vi "运维调试_总磷氨氮.vi"() -> ()   [LabVIEW 2016, in "斯坦道仪器.lvlib"]
uses:
  <vilib>/Platform/TimedLoop/XDataNode/timing_clust.ctl
  <vilib>/Platform/TimedLoop/XDataNode/nitl_modes.ctl
  <vilib>/Platform/TimedLoop/XDataNode/wakeup.ctl
  <vilib>/Utility/miscctls.llb/LVPointTypeDef.ctl
  <vilib>/Platform/TimedLoop/XDataNode/XDataNode.xnode
  <vilib>/Platform/TimedLoop/XDataNode/XDNodeRunTimeDep.lvlib
panel:
  out "固件版本号":string
  in  "参数":T1={"站号"=3, "量程切换"=enum."AUTO", "控制命令"=enum."启动测量", "模式设置"=enum."待机", "测量间隔"=0} {"站号" items=["氨氮"=3]}
  out "error out":errorcluster
  in  "同步时间":bool
  in  "数组":string[](array[string])
  in  "备用系数写入":bool
  in  "备用系数读取":bool
  in  "备用系数":T2
  in  "量程切换阈值写入":bool
  in  "量程切换阈值读取":bool
  in  "量程切换阈值":cluster{"阈值":dbl, "标液浓度":dbl}
  in  "参数下拉列表":enum16{"氨氮"}(ring)
  in  "量程下拉列表":enum16{"低量程", "高量程"}(ring)
  in  "测量模式下拉列表":enum16{"水样测量", "空白核查", "标样核查", "盲样测试", "加标回收"}(ring)
  in  "公式":cluster{"X^2":dbl, "X":dbl, "b":dbl}
  in  "写公式":bool
  in  "读公式":bool
  in  "精度":dbl=4.0
  in  "样品5 F0":dbl
  in  "样品5 F1":dbl
  in  "样品4 F1":dbl
  in  "样品4 F0":dbl
  in  "样品3 F0":dbl
  in  "样品3 F1":dbl
  in  "样品2 F0":dbl
  in  "样品2 F1":dbl
  in  "样品1 F1":dbl
  in  "样品1 F0":dbl
  in  "method":u16(ring) items=["最小二乘", "最小绝对残差", "Bisquare"]
  in  "模型":enum32{"线性", "多项式"}(ring)
  out "r^2":dbl format="%.7g"
  out "拟合公式":string
  in  "样品2启用":bool
  in  "样品5启用":bool
  in  "样品4启用":bool
  in  "样品3启用":bool
  in  "样品1启用":bool
  in  "标液浓度5":dbl
  out "测量吸光度5":dbl
  in  "标液浓度4":dbl
  out "测量吸光度4":dbl
  in  "标液浓度3":dbl
  out "测量吸光度3":dbl
  in  "标液浓度2":dbl
  out "测量吸光度2":dbl
  out "测量吸光度1":dbl
  in  "标液浓度1":dbl
  out "XY图":cluster{"X Values":dbl[], "Y Values":dbl[]}[](graph)
  in  "返回":bool
  in  "设置":bool
  out "序列号":string="序列号"
  out "氨氮测量数据":T3(xcontrol)
  out "总磷测量数据":T3(xcontrol)
  out "集成报警信息":string
  out "设置值":dbl
  out "定时启动":bool
  out "总磷总氮运行状态":T4(xcontrol)
  in  "停止":bool
  in  "手动启动":bool
  in  "单步测试":bool
  in  "总磷氨氮调试":u16[](xcontrol)
  out "F3":sgl format="%#.6f"
  out "F2":sgl format="%#.6f"
  out "F1":sgl format="%#.6f"
  out "F0":sgl format="%#.6f"
  out "多列列表框":i32(listbox)
  # "COM4"
  # "参数设置"
  # "标液浓度"
  # "F0"
  # "F1"
  # "吸光值显示"
  # "样品一"
  # "辅\n助\n计\n算\n区"
  # "样品二"
  # "样品三"
  # "样品四"
  # "样品五"
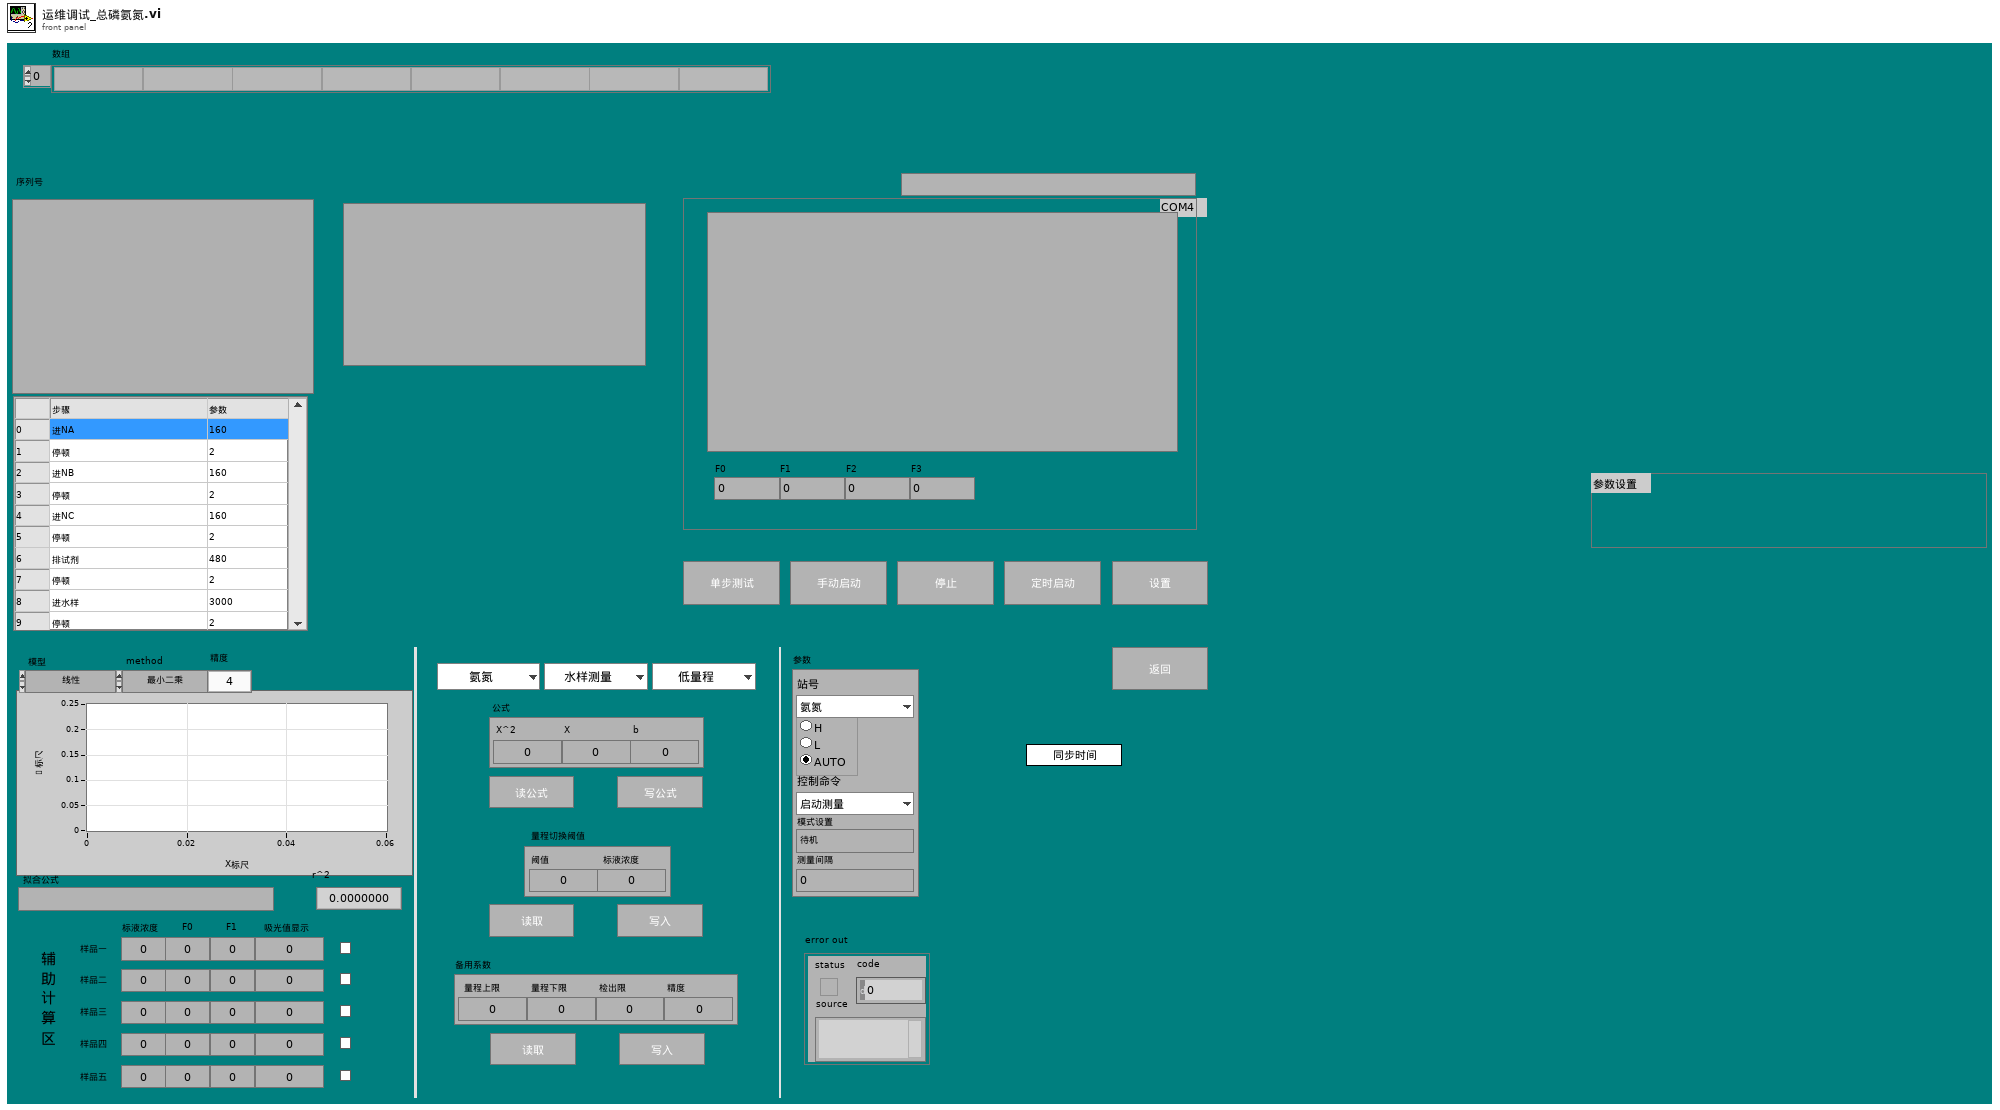
[diagram p1: front panel]
types:
  T1 = cluster{"站号":u16, "量程切换":enum32{"H", "L", "AUTO"}, "控制命令":enum16{"启动测量", "标样核查", "零点核查", "跨度核查", "空白测试", "平行样测试", "加标回收", "空白校准", "标样校准", "初始化（清洗）", "停止测试", "仪器重启", "校时", "模式设置", "测量间隔设置", ""}, "模式设置":enum16{"待机", "连续模式", "周期模式", "定点模式", "受控模式", "手动模式"}, "测量间隔":u16}
  T2 = cluster{"量程上限":dbl, "量程下限":dbl, "检出限":dbl, "精度":dbl}
  T3 = cluster{"flowid":u16, "测量精度":u16, "测量数据区":cluster{"因子编码":u32, "单位":u16, "标样参考值":sgl, "水样数据时间":timestamp, "水样实测值":sgl, "水样数据标识":string, "标样数据时间":timestamp, "标样实测值":sgl, "标样数据标识":string, "空白数据时间":timestamp, "空白实测值":sgl, "空白数据标识":string, "零点核查数据时间":timestamp, "零点核查实测值":sgl, "零点核查数据标识":string, "跨度核查数据时间":timestamp, "跨度核查实测值":sgl, "跨度核查数据标识":string, "加标回收数据时间":timestamp, "加标回收实测值":sgl, "加标回收数据标识":string, "平行样数据时间":timestamp, "平行样实测值":sgl, "平行样数据标识":string}}
  T4 = cluster{"系统时间":timestamp, "工作状态":enum16{"空闲", "水样测试", "标样核查", "零点核查", "跨度核查", "空白测试", "平行样测试", "加标回收", "空白校准", "标样校准", "初始化（清洗）"}, "测量模式":enum16{"待机", "连续模式", "周期模式", "定点模式", "受控模式", "手动模式"}, "告警代码":enum16{"无告警", "缺试剂告警", "缺水样告警", "缺蒸馏水告警", "缺标液告警", "仪表漏液告警", "标定异常告警", "超量程告警", "加热异常", "低试剂预警", "超上限告警", "超下限告警", "仪表内部其他异常", "滴定异常告警", "电极异常告警", "量程切换告警", "参数设置告警", "PH电极电位异常", "电导率电极异常", "浊度光度异常", "溶解氧电极异常", "溶解氧光强异常", "温度异常告警", "PH异常告警", "溶解氧异常告警", "电导率异常告警", "浊度异常告警", "叶绿素异常告警", "藻密度异常告警", "蓝绿藻异常告警", "ORP异常告警", "氨氮异常告警", "清洁刷异常告警", "SD卡异常告警", "蓝牙异常告警", "Wifi异常告警", "流程异常告警"}, "故障代码":enum16{"无故障", "电机故障", "温度故障", "通讯故障", "滴定故障"}, "日志代码":u16, "软件版本":u16, "F0":sgl, "F1":sgl, "F2":sgl, "F3":sgl, "T":sgl, "H":sgl, "id":u16, "flowid":u16, "量程":u16}
  T5 = enum16{"待机", "启动氨氮", "氨氮测量中", "启动总磷", "总磷测量中", "延时"}
  T6 = typedef "LVPointTypeDef.ctl" = cluster{"Horizontal":i16, "Vertical":i16}
  T7 = cluster{"因子编码":u32, "单位":u16, "标样参考值":sgl, "水样数据时间":timestamp, "水样实测值":sgl, "水样数据标识":string, "标样数据时间":timestamp, "标样实测值":sgl, "标样数据标识":string, "空白数据时间":timestamp, "空白实测值":sgl, "空白数据标识":string, "零点核查数据时间":timestamp, "零点核查实测值":sgl, "零点核查数据标识":string, "跨度核查数据时间":timestamp, "跨度核查实测值":sgl, "跨度核查数据标识":string, "加标回收数据时间":timestamp, "加标回收实测值":sgl, "加标回收数据标识":string, "平行样数据时间":timestamp, "平行样实测值":sgl, "平行样数据标识":string}
  T8 = enum16{"空闲", "水样测试", "标样核查", "零点核查", "跨度核查", "空白测试", "平行样测试", "加标回收", "空白校准", "标样校准", "初始化（清洗）"}
  T9 = cluster{"启动模式":enum16{"标液测量", "水样测量", "零液测量", "盲样测量", "加标回收"}, "启动参数":u16, "量程":enum16{"低量程", "高量程"}}
  T10 = cluster{"时间标识":timestamp, "设备":string, "日志信息":string, "流程参数":string}
  T11 = cluster{"时间标识":timestamp, "设备":string, "日志信息":string}
  T12 = enum16{"无告警", "缺试剂告警", "缺水样告警", "缺蒸馏水告警", "缺标液告警", "仪表漏液告警", "标定异常告警", "超量程告警", "加热异常", "低试剂预警", "超上限告警", "超下限告警", "仪表内部其他异常", "滴定异常告警", "电极异常告警", "量程切换告警", "参数设置告警", "PH电极电位异常", "电导率电极异常", "浊度光度异常", "溶解氧电极异常", "溶解氧光强异常", "温度异常告警", "PH异常告警", "溶解氧异常告警", "电导率异常告警", "浊度异常告警", "叶绿素异常告警", "藻密度异常告警", "蓝绿藻异常告警", "ORP异常告警", "氨氮异常告警", "清洁刷异常告警", "SD卡异常告警", "蓝牙异常告警", "Wifi异常告警", "流程异常告警"}
  T13 = typedef "LVRowAndColumnUnsignedTypeDef.ctl" = cluster{"Row":u32, "Column":u32}
  T14 = typedef "XDNodeRunTimeDep.lvlib/timing_clust.ctl" = cluster{"Expected End [f-1]":u64, "Actual End [f-1]":u64, "Finished Late? [f-1]":bool, "Expected End [i-1]":u64, "Actual End [i-1]":u64, "Finished Late? [i-1]":bool, "Expected Start [i]":u64, "Actual Start [i]":u64, "Expected Start [f]":u64, "Actual Start [f]":u64, "Source Name":string, "Structure Name":string, "Period":i64, "Deadline":i64, "Offset":i64, "Start":i64, "Priority":i32, "Timeout":i32, "Mode":T15, "Wakeup Reason":T16, "Error":errorcluster, "Source Type":string, "Secondary Source Type":string, "Global End Time":u64, "Global Start Time":u64, "Frame Duration":u64, "Iteration Duration":u64, "Assigned CPU":i32, "I/O Scan Engine Mode":u32}
  T15 = typedef "XDNodeRunTimeDep.lvlib/nitl_modes.ctl" = enum32{"No Change", "Process missed periods, maintain original phase", "Discard missed periods, maintain original phase", "Process missed periods, ignore original phase", "Discard missed periods, ignore original phase"}
  T16 = typedef "XDNodeRunTimeDep.lvlib/wakeup.ctl" = enum32{"Normal", "Aborted", "Asynchronous wakeup", "Timing source error", "Timed loop error", "Timeout"}
  T17 = cluster{"站号":u16, "量程切换":enum32{"H", "L", "AUTO"}, "控制命令":enum16{"启动测量", "标样核查", "零点核查", "跨度核查", "空白测试", "平行样测试", "加标回收", "空白校准", "标样校准", "初始化（清洗）", "停止测试", "仪器重启", "校时", "模式设置", "测量间隔设置", "盲样测试"}, "模式设置":enum16{"待机", "连续模式", "周期模式", "定点模式", "受控模式", "手动模式"}, "测量间隔":u16}
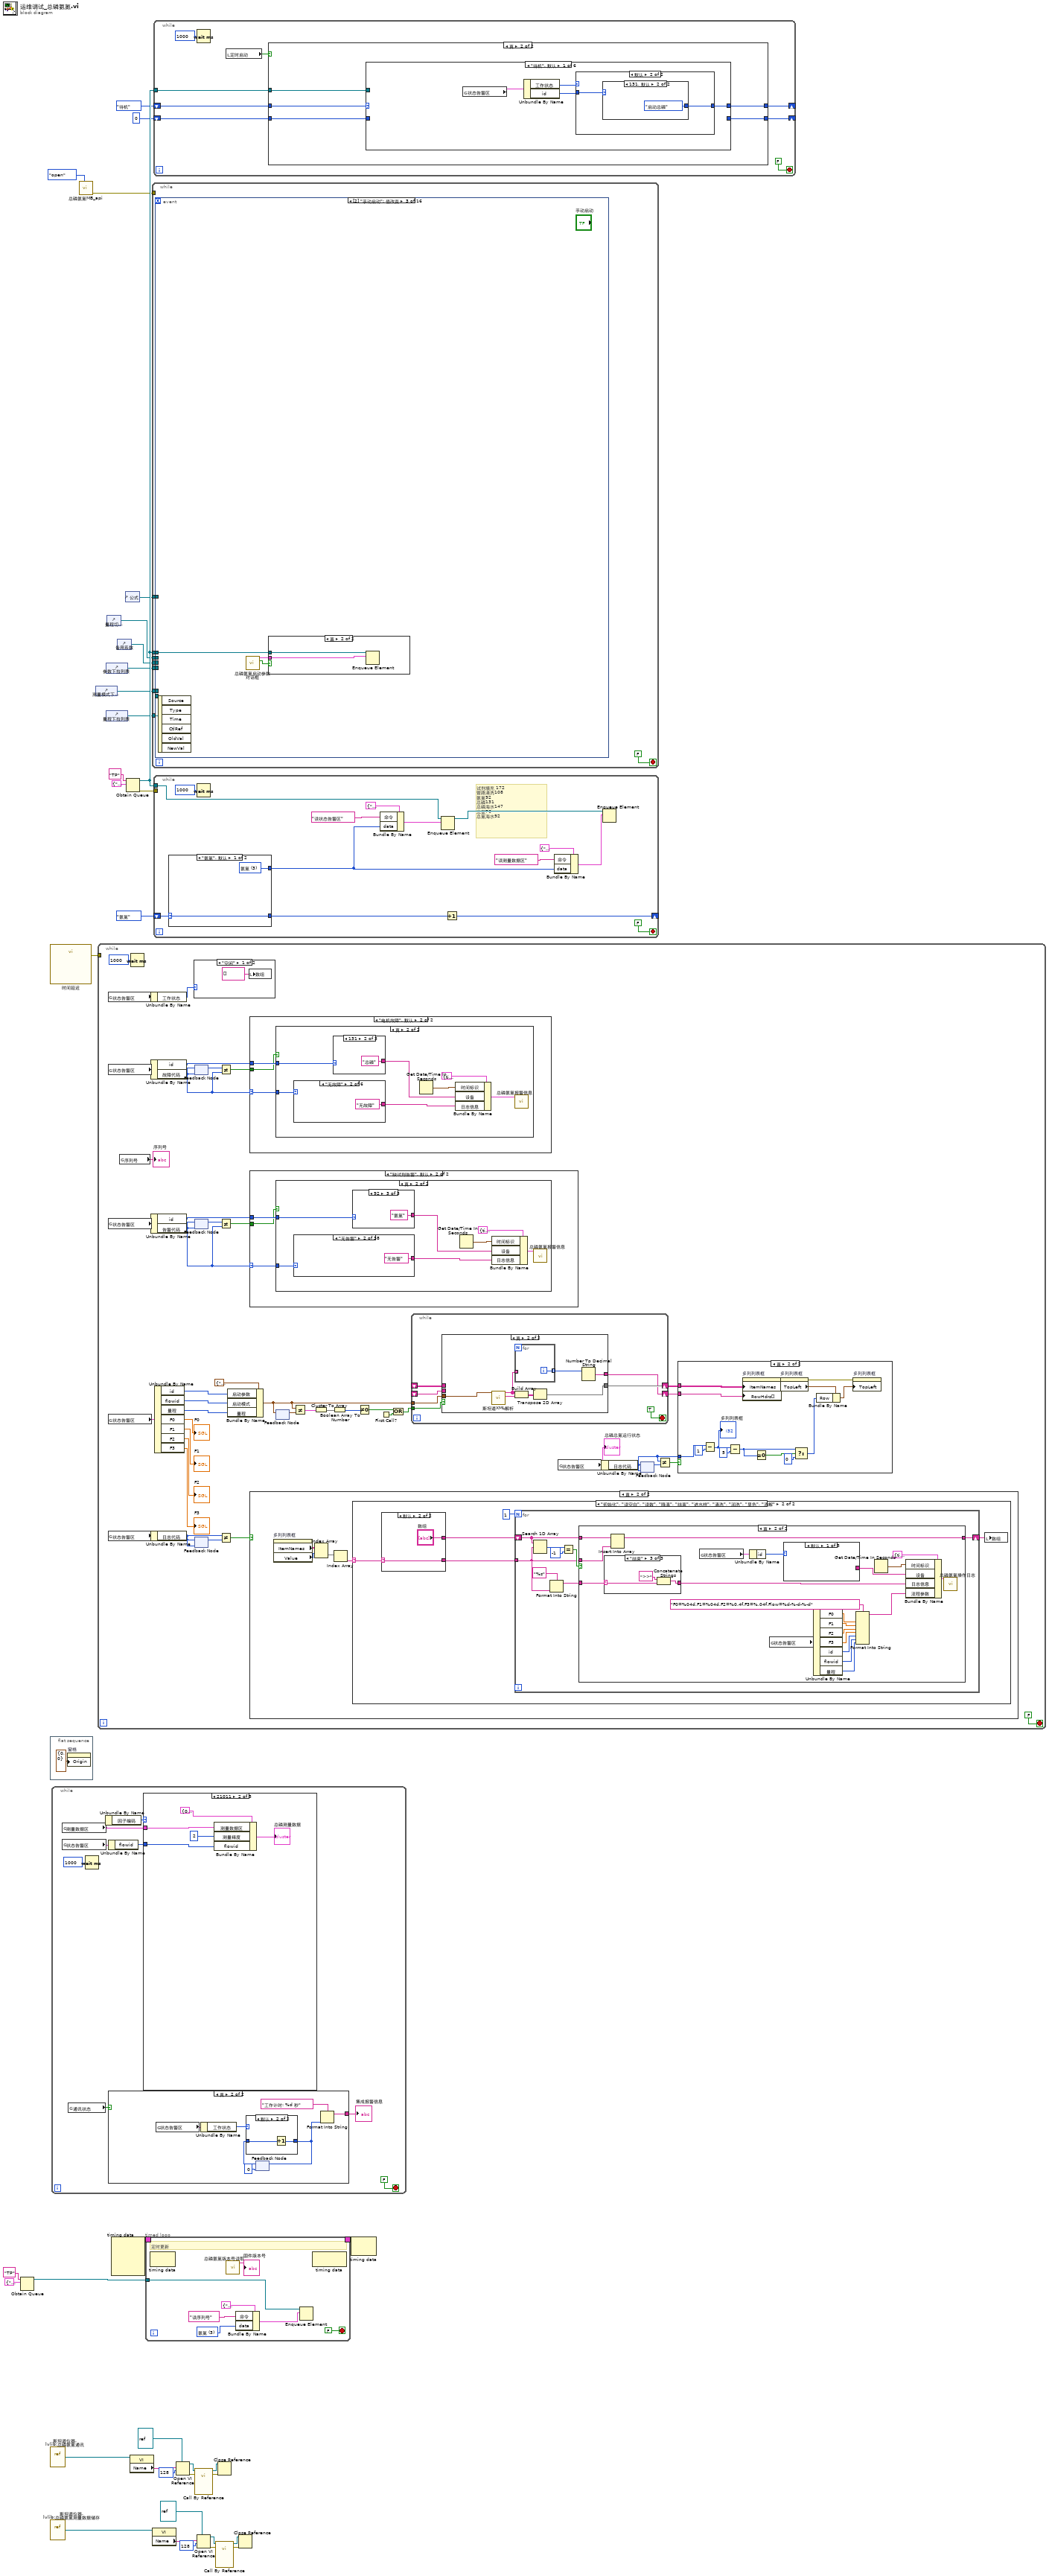
[diagram p0: block diagram]
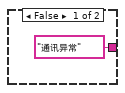
[diagram p2: hidden frame]
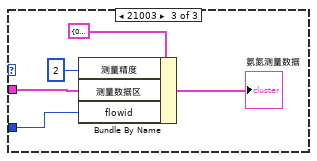
[diagram p5: hidden frame]
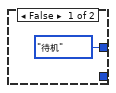
[diagram p6: hidden frame]
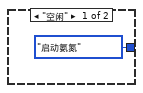
[diagram p7: hidden frame]
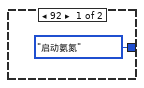
[diagram p8: hidden frame]
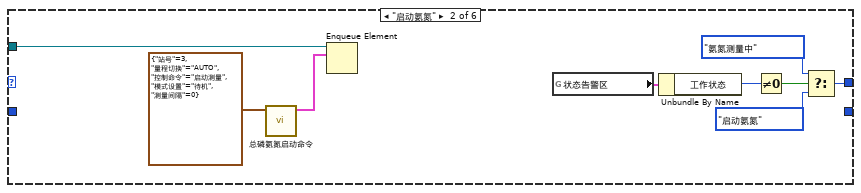
[diagram p9: hidden frame]
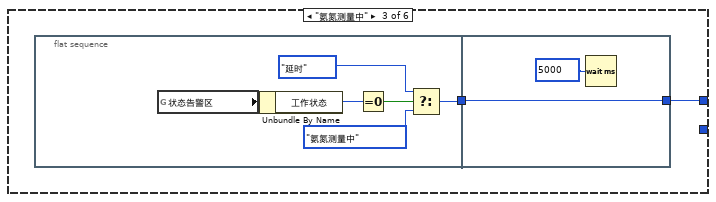
[diagram p10: hidden frame]
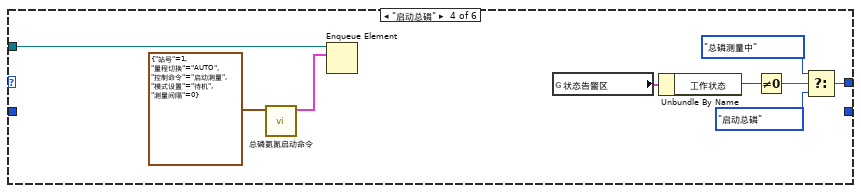
[diagram p11: hidden frame]
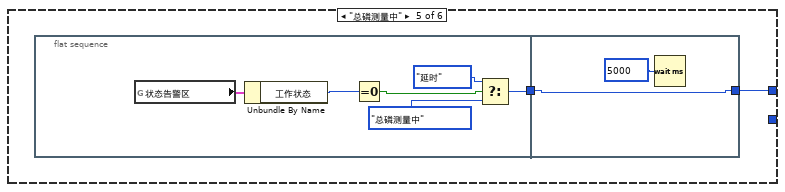
[diagram p12: hidden frame]
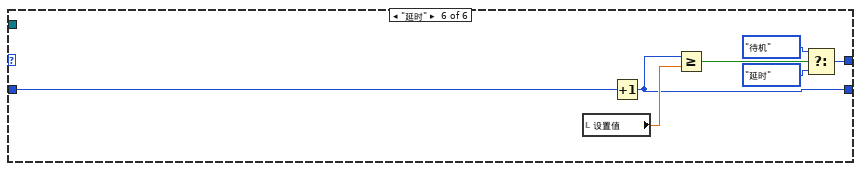
[diagram p13: hidden frame]
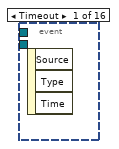
[diagram p14: hidden frame]
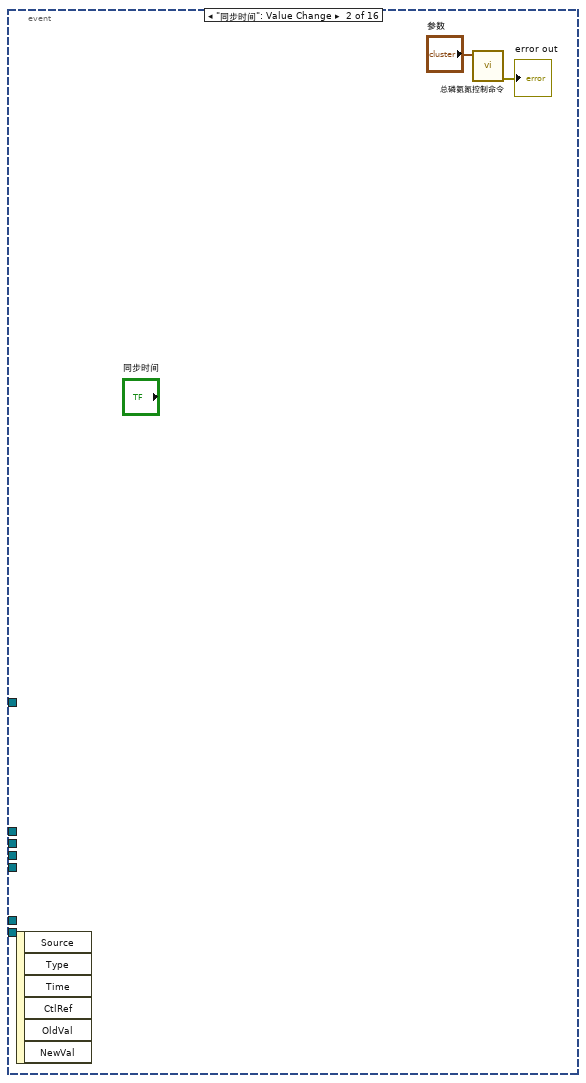
[diagram p15: hidden frame]
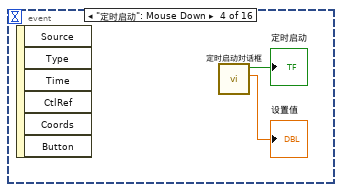
[diagram p17: hidden frame]
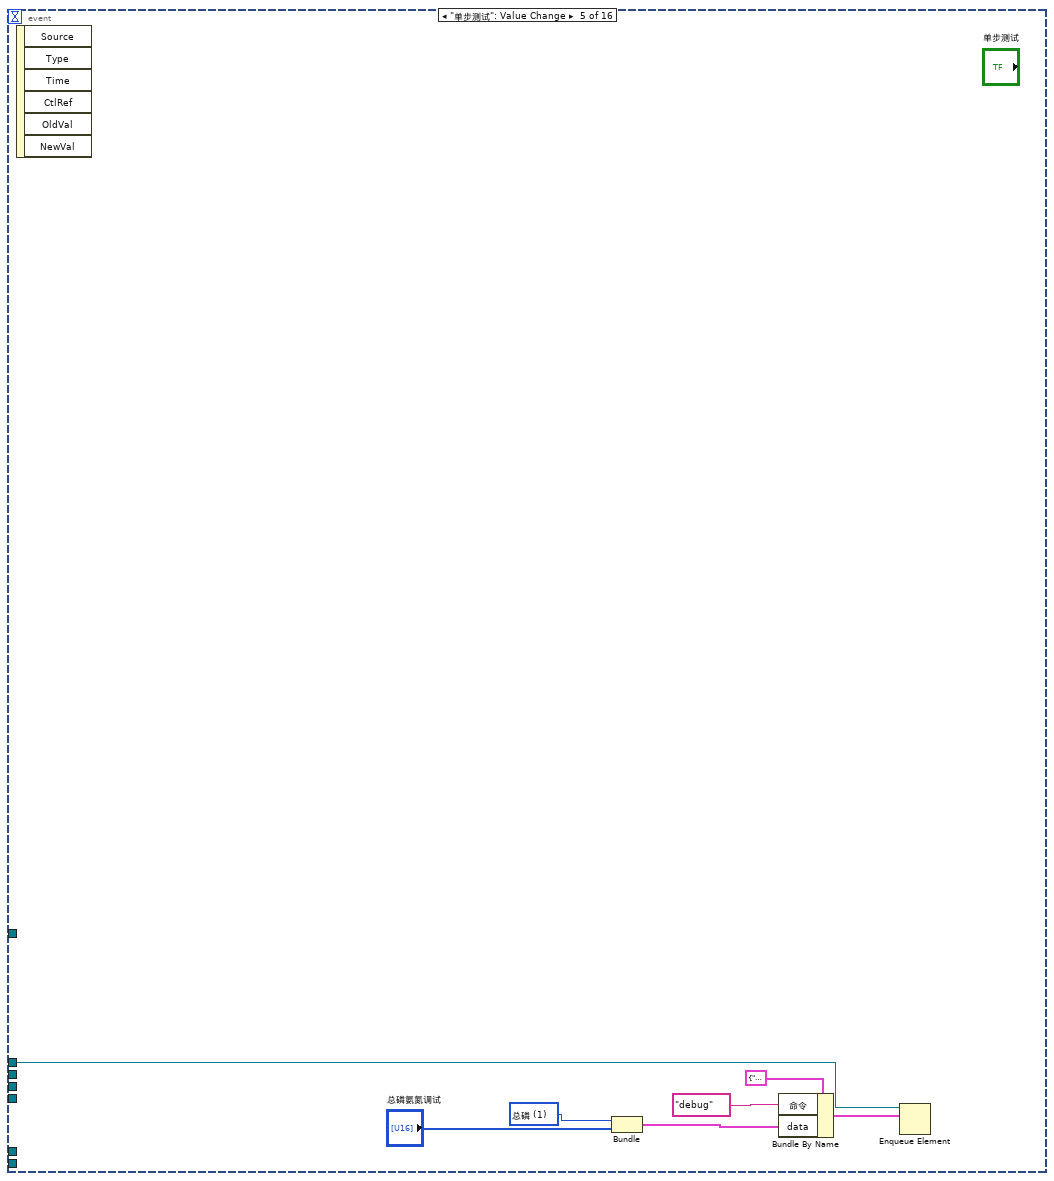
[diagram p18: hidden frame]
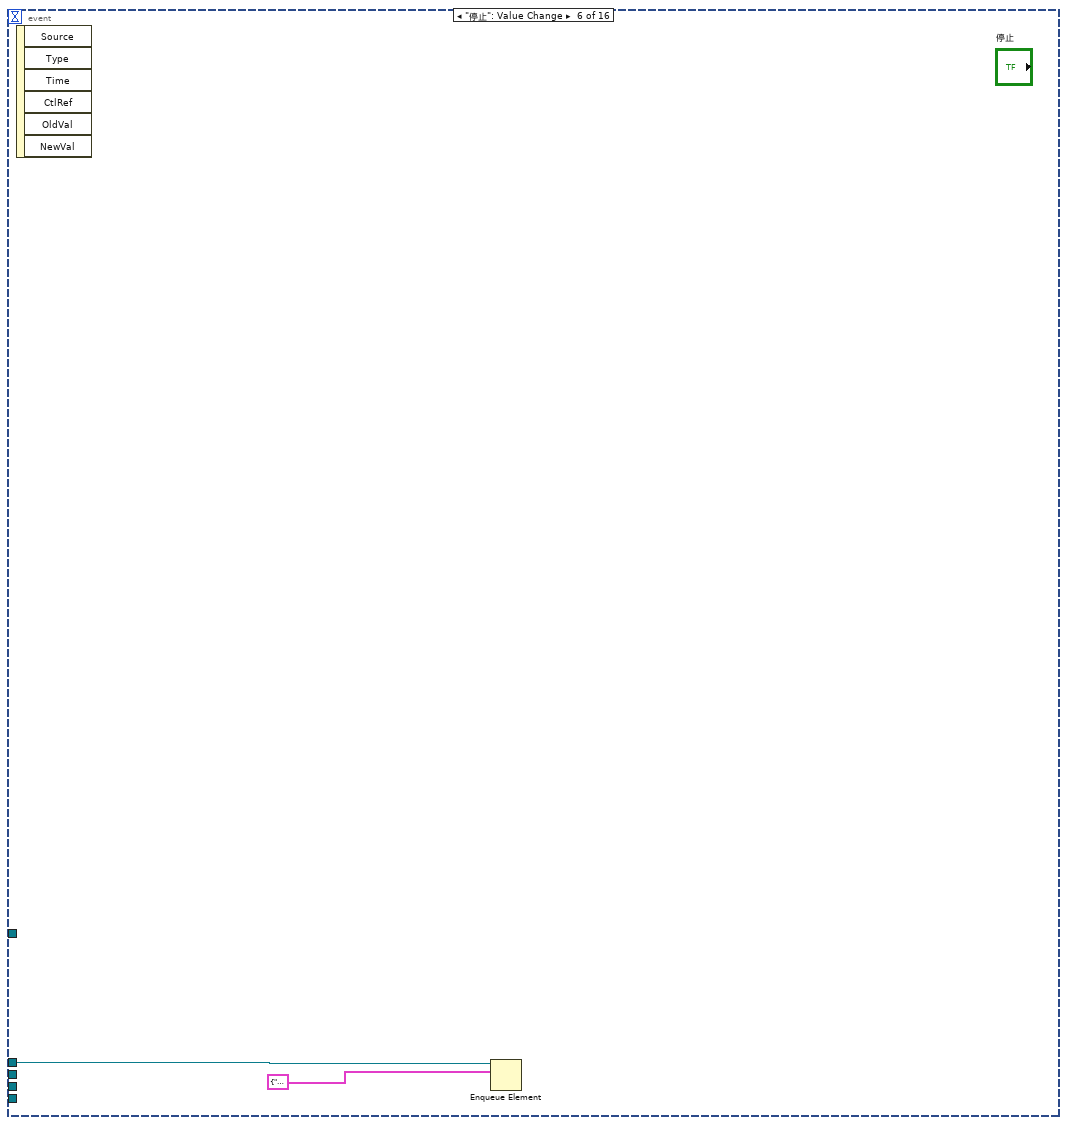
[diagram p19: hidden frame]
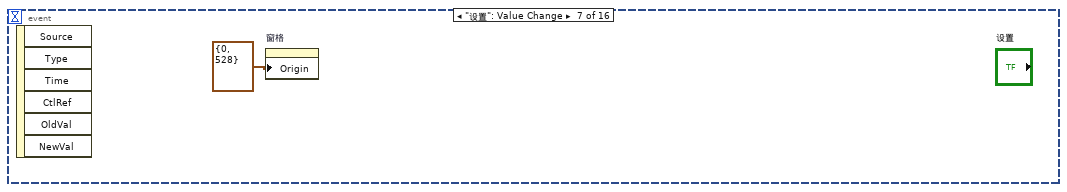
[diagram p20: hidden frame]
diagram:
  n1 = Obtain Queue(name (unnamed)="TP" ("名称（未命名）"), element data type=cluster{"命令":string, "data":variant} {"命令"="", "data"=variant}) -> (queue out=w1:refnum<queue>)  [unwired: 3 in, 2 out]
  n2 = call "时间延迟"() -> ("error out"=w8:errorcluster)  [unwired: 11 in]
  n3 = flat-sequence {
    frame #0 {
      n4 = property on="窗格" class="Pane"("Origin"=T6 {"Horizontal"=0, "Vertical"=0} ("原点")) -> ()  [unwired: 2 in, 2 out]
    }
  }
  n5 = vi-ref "斯坦道仪器.lvlib:总磷氨氮通讯.vi"() -> (w31:refnum<vi>)
  n6 = vi-ref "斯坦道仪器.lvlib:总磷氨氮测量数据储存.vi"() -> (w23:refnum<vi>)
  n7 = while {
    stop <- FALSE stop-if-true
    n8 = global read "VAR总磷氨氮全局变量.vi" "测量数据区"() -> (w44:T7)
    n9 = global read "VAR总磷氨氮全局变量.vi" "状态告警区"() -> (w40:T4)
    n10 = global read "VAR总磷氨氮全局变量.vi" "通讯状态"() -> (w42:bool)
    n11 = Wait (ms)(milliseconds to wait=u32 1000 ("等待时间（毫秒）")) -> ()  [unwired: 1 out]
    n12 = Unbundle By Name(w44) -> ("因子编码"=w43:u32)
    n13 = case shown="真" w42 {
      tunnel: ["通讯异常" ("集成报警信息") w48] -> w41
      frame False {
      }
      frame True {
        n14 = global read "VAR总磷氨氮全局变量.vi" "状态告警区"() -> (w54:T4)
        n15 = Unbundle By Name(w54) -> ("工作状态"=w53:T8)
        n16 = feedback #1(0) -> (w51:i32)
        n17 = case shown="默认" w53 {
          tunnel: w51 -> [_ w56]
          tunnel: [_ w55] -> w49
          frame "空闲" {
          }
          frame Default {
            n18 = Increment(x=w56) -> (x+1=w55:i32)
          }
        }
        n19 = feedback-in #1(w49) -> ()
        n20 = Format Into String(format string="工作计时: %d 秒" ("格式字符串"), w49) -> (resulting string=w48:string)  [unwired: 2 in, 1 out]
      }
    }
    "集成报警信息" <- w41
    n21 = Unbundle By Name(w40) -> ("flowid"=w39:u16)
    n22 = case shown="21011" w43 {
      tunnel: w44 -> [_ w61 w66]
      tunnel: w39 -> [_ w58 w64]
      frame Default {
      }
      frame 21011 {
        n23 = Bundle By Name(cluster=T3 {"flowid"=0, "测量精度"=0, "测量数据区"={"因子编码"=0, "单位"=0, "标样参考值"=0.0, "水样数据时间"=timestamp(0 s since 1904-01-01), "水样实测值"=0.0, "水样数据标识"="", "标样数据时间"=timestamp(0 s since 1904-01-01), "标样实测值"=0.0, "标样数据标识"="", "空白数据时间"=timestamp(0 s since 1904-01-01), "空白实测值"=0.0, "空白数据标识"="", "零点核查数据时间"=timestamp(0 s since 1904-01-01), "零点核查实测值"=0.0, "零点核查数据标识"="", "跨度核查数据时间"=timestamp(0 s since 1904-01-01), "跨度核查实测值"=0.0, "跨度核查数据标识"="", "加标回收数据时间"=timestamp(0 s since 1904-01-01), "加标回收实测值"=0.0, "加标回收数据标识"="", "平行样数据时间"=timestamp(0 s since 1904-01-01), "平行样实测值"=0.0, "平行样数据标识"=""}} ("氨氮测量数据"), "测量数据区"=w61, "测量精度"=u16 2, "flowid"=w58) -> (→"总磷测量数据":T3)
      }
      frame 21003 {
        n24 = Bundle By Name(cluster=T3 {"flowid"=0, "测量精度"=0, "测量数据区"={"因子编码"=0, "单位"=0, "标样参考值"=0.0, "水样数据时间"=timestamp(0 s since 1904-01-01), "水样实测值"=0.0, "水样数据标识"="", "标样数据时间"=timestamp(0 s since 1904-01-01), "标样实测值"=0.0, "标样数据标识"="", "空白数据时间"=timestamp(0 s since 1904-01-01), "空白实测值"=0.0, "空白数据标识"="", "零点核查数据时间"=timestamp(0 s since 1904-01-01), "零点核查实测值"=0.0, "零点核查数据标识"="", "跨度核查数据时间"=timestamp(0 s since 1904-01-01), "跨度核查实测值"=0.0, "跨度核查数据标识"="", "加标回收数据时间"=timestamp(0 s since 1904-01-01), "加标回收实测值"=0.0, "加标回收数据标识"="", "平行样数据时间"=timestamp(0 s since 1904-01-01), "平行样实测值"=0.0, "平行样数据标识"=""}} ("氨氮测量数据"), "测量精度"=u16 2, "测量数据区"=w66, "flowid"=w64) -> (→"氨氮测量数据":T3)
      }
    }
  }
  n25 = call "总磷氨氮MB_api.vi"("STEP"=enum16{"open", "read", "write", "close"}."open") -> ("error out"=w7:errorcluster)  [unwired: 8 in, 2 out]
  n26 = control-ref of="测量模式下拉列表"() -> (w12:refnum<vi>)
  n27 = while {
    tunnel: w8 -> [_]
    stop <- FALSE stop-if-true
    n28 = global read "VAR总磷氨氮全局变量.vi" "状态告警区"() -> (w72:T4)
    n29 = global read "VAR总磷氨氮全局变量.vi" "状态告警区"() -> (w78:T4)
    n30 = global read "VAR总磷氨氮全局变量.vi" "状态告警区"() -> (w83:T4)
    n31 = global read "VAR总磷氨氮全局变量.vi" "状态告警区"() -> (w95:T4)
    n32 = global read "VAR总磷氨氮全局变量.vi" "状态告警区"() -> (w69:T4)
    n33 = global read "VAR总磷氨氮全局变量.vi" "序列号"() -> (→"序列号":string)
    n34 = Wait (ms)(milliseconds to wait=u32 1000 ("等待时间（毫秒）")) -> ()  [unwired: 1 out]
    n35 = Unbundle By Name(w72) -> ("工作状态"=w71:T8)
    n36 = Unbundle By Name(w78) -> ("id"=w77:u16, "故障代码"=w74:enum16{"无故障", "电机故障", "温度故障", "通讯故障", "滴定故障"})
    n37 = Unbundle By Name(w83) -> ("id"=w82:u16, "告警代码"=w79:T12)
    n38 = Unbundle By Name(w69) -> ("日志代码"=w68:u16)
    n39 = Unbundle By Name(w95) -> ("id"=w92:u16, "flowid"=w94:u16, "量程"=w93:u16, "F0"=→"F0":sgl, "F1"=→"F1":sgl, "F2"=→"F2":sgl, "F3"=→"F3":sgl)
    n40 = case shown="\"空闲\"" w71 {
      frame "空闲" {
        n41 = local write "数组"(string[] [] ("数组")) -> ()
      }
      frame "水样测试", Default {
      }
    }
    n42 = feedback #2(w74) -> (w75:enum16{"无故障", "电机故障", "温度故障", "通讯故障", "滴定故障"})
    n43 = feedback-in #2(w74) -> ()
    n44 = feedback #3(w79) -> (w80:T12)
    n45 = feedback-in #3(w79) -> ()
    n46 = feedback #4(w68) -> (w70:u16)
    n47 = feedback-in #4(w68) -> ()
    n48 = Not Equal?(x=w75, y=w74) -> (x != y?=w76:bool)
    n49 = Not Equal?(x=w80, y=w79) -> (x != y?=w81:bool)
    n50 = Not Equal?(x=w68, y=w70) -> (x != y?=w67:bool)
    n51 = Bundle By Name(cluster=T9 {"启动模式"=enum."加标回收", "启动参数"=1, "量程"=enum."低量程"} ("参数簇"), "启动参数"=w92, "启动模式"=w94, "量程"=w93) -> (w85:T9)
    n52 = case shown="\"电机故障\", 默认" w74 {
      selector: w74 -> [_ w163]
      tunnel: w77 -> [_ w164]
      tunnel: w76 -> [_ w162]
      frame "无故障" {
      }
      frame "电机故障", Default {
        n53 = case shown="真" w162 {
          tunnel: w164 -> [_ w171]
          tunnel: w163 -> [_ w166]
          frame False {
          }
          frame True {
            n54 = case shown="\"无故障\"" w166 {
              selector: w166 -> [w173 _ _ _ _ _]
              tunnel: [w172 "无故障" "电机故障" "温度故障" "通讯故障" "滴定故障"] -> w165
              frame Default {
                n55 = Format Into String(format string="%d" ("格式字符串"), initial string="未知" ("工作状态"), w173) -> (resulting string=w172:string)  [unwired: 1 in, 1 out]
              }
              frame "无故障" {
              }
              frame "电机故障" {
              }
              frame "温度故障" {
              }
              frame "通讯故障" {
              }
              frame "滴定故障" {
              }
            }
            n56 = case shown="131" w171 {
              tunnel: [_ "总磷" ("table输入") "氨氮" ("table输入")] -> w167
              frame Default {
              }
              frame 131 {
              }
              frame 92 {
              }
            }
            n57 = Get Date/Time In Seconds() -> (seconds since 1Jan1904=w168:timestamp)
            n58 = Bundle By Name(cluster=T11 {"时间标识"=timestamp(0 s since 1904-01-01), "设备"="", "日志信息"=""} ("data in"), "时间标识"=w168, "设备"=w167, "日志信息"=w165) -> (w169:T11)
            n59 = call "总磷氨氮报警信息.vi"("data in"=w169) -> ()  [unwired: 11 in]
          }
        }
      }
    }
    n60 = case shown="\"缺试剂告警\", 默认" w79 {
      selector: w79 -> [_ w184]
      tunnel: w82 -> [_ w185]
      tunnel: w81 -> [_ w183]
      frame "无告警" {
      }
      frame "缺试剂告警", Default {
        n61 = case shown="真" w183 {
          tunnel: w185 -> [_ w192]
          tunnel: w184 -> [_ w186]
          frame False {
          }
          frame True {
            n62 = case shown="\"无告警\"" w186 {
              selector: w186 -> [w194 _ _ _ _ _ _ _ _ _ _ _ _ _ _ _ _ _ _ _ _ _ _ _ _ _ _ _ _ _ _ _ _ _ _ _ _ _]
              tunnel: [w193 "无告警" "缺试剂告警" "缺水样告警" "缺蒸馏水告警" "缺标液告警" "仪表漏液告警" "标定异常告警" "超量程告警" "加热异常" "低试剂预警" "超上限告警" "超下限告警" "仪表内部其他异常" "滴定异常告警" "电极异常告警" "量程切换告警" "参数设置告警" "PH电极电位异常" "电导率电极异常" "浊度光度异常" "溶解氧电极异常" "溶解氧光强异常" "温度异常告警" "PH异常告警" "溶解氧异常告警" "电导率异常告警" "浊度异常告警" "叶绿素异常告警" "藻密度异常告警" "蓝绿藻异常告警" "ORP异常告警" "氨氮异常告警" "清洁刷异常告警" "SD卡异常告警" "蓝牙异常告警" "WiFi异常告警" "流程异常告警"] -> w187
              frame Default {
                n63 = Format Into String(format string="%d" ("格式字符串"), initial string="未知" ("工作状态"), w194) -> (resulting string=w193:string)  [unwired: 1 in, 1 out]
              }
              frame "无告警" {
              }
              frame "缺试剂告警" {
              }
              frame "缺水样告警" {
              }
              frame "缺蒸馏水告警" {
              }
              frame "缺标液告警" {
              }
              frame "仪表漏液告警" {
              }
              frame "标定异常告警" {
              }
              frame "超量程告警" {
              }
              frame "加热异常" {
              }
              frame "低试剂预警" {
              }
              frame "超上限告警" {
              }
              frame "超下限告警" {
              }
              frame "仪表内部其他异常" {
              }
              frame "滴定异常告警" {
              }
              frame "电极异常告警" {
              }
              frame "量程切换告警" {
              }
              frame "参数设置告警" {
              }
              frame "PH电极电位异常" {
              }
              frame "电导率电极异常" {
              }
              frame "浊度光度异常" {
              }
              frame "溶解氧电极异常" {
              }
              frame "溶解氧光强异常" {
              }
              frame "温度异常告警" {
              }
              frame "PH异常告警" {
              }
              frame "溶解氧异常告警" {
              }
              frame "电导率异常告警" {
              }
              frame "浊度异常告警" {
              }
              frame "叶绿素异常告警" {
              }
              frame "藻密度异常告警" {
              }
              frame "蓝绿藻异常告警" {
              }
              frame "ORP异常告警" {
              }
              frame "氨氮异常告警" {
              }
              frame "清洁刷异常告警" {
              }
              frame "SD卡异常告警" {
              }
              frame "蓝牙异常告警" {
              }
              frame "Wifi异常告警" {
              }
              frame "流程异常告警" {
              }
            }
            n64 = case shown="92" w192 {
              tunnel: [_ "总磷" ("table输入") "氨氮" ("table输入")] -> w188
              frame Default {
              }
              frame 131 {
              }
              frame 92 {
              }
            }
            n65 = Get Date/Time In Seconds() -> (seconds since 1Jan1904=w189:timestamp)
            n66 = Bundle By Name(cluster=T11 {"时间标识"=timestamp(0 s since 1904-01-01), "设备"="", "日志信息"=""} ("data in"), "时间标识"=w189, "设备"=w188, "日志信息"=w187) -> (w190:T11)
            n67 = call "总磷氨氮报警信息.vi"("data in"=w190) -> ()  [unwired: 11 in]
          }
        }
      }
    }
    n68 = case shown="真" w67 {
      frame False {
      }
      frame True {
        n69 = property on="多列列表框" class="MCListbox (严格)"() -> ("ItemNames"=w112:string[][], "Value"=w113:i32)  [unwired: 2 in, 2 out]
        n70 = Index Array(array=w112, index (row)=w113) -> (element=w111:string[])  [unwired: 1 in]
        n71 = Index Array(array=w111) -> (element=w110:string)  [unwired: 1 in]
        n72 = case shown="\"初始化\", \"读空白\", \"读数\", \"降温\", \"结束\", \"进水样\", \"清洗\", \"润洗\", \"显色\", \"消解\"" w110 {
          selector: w110 -> [_ w116]
          frame Default {
          }
          frame "初始化", "读空白", "读数", "降温", "结束", "进水样", "清洗", "润洗", "显色", "消解" {
            n73 = case shown="默认" w116 {
              selector: w116 -> [w120 w122]
              tunnel: [w120 w122] -> w115
              tunnel: [string[] [] ("数组") "数组"] -> w114
              frame "读数" {
              }
              frame Default {
              }
            }
            n74 = for {
              N: 1 -> [_]
              tunnel: w115 -> [w124]
              shift-right: [w123] -> w117
              shift-left: w114 -> [w125]
              n75 = Search 1D Array(1D array=w125, element=w124) -> (index of element=w128:i32)  [unwired: 1 in]
              n76 = Format Into String(format string="%s" ("格式字符串"), w124) -> (resulting string=w129:string)  [unwired: 2 in, 1 out]
              n77 = Equal?(x=w128, y=-1) -> (x = y?=w126:bool)
              n78 = case shown="真" w126 {
                tunnel: w129 -> [_ w133]
                tunnel: w125 -> [w131 w137]
                tunnel: w124 -> [_ w136]
                tunnel: [w131 w135] -> w123
                frame False {
                }
                frame True {
                  n79 = case shown="\"结束\"" w133 {
                    selector: w133 -> [w153 w156 w159]
                    tunnel: [w153 w155 w158] -> w132
                    frame Default {
                    }
                    frame "初始化" {
                      n80 = Concatenate Strings("<<" ("字符串"), w156) -> (w155:string)
                    }
                    frame "结束" {
                      n81 = Concatenate Strings(">>" ("字符串"), w159) -> (w158:string)
                    }
                  }
                  n82 = Insert Into Array(array=w137, new element=w136) -> (w135:string[])  [unwired: 1 in]
                  n83 = global read "VAR总磷氨氮全局变量.vi" "状态告警区"() -> (w152:T4)
                  n84 = Unbundle By Name(w152) -> ("id"=w151:u16)
                  n85 = global read "VAR总磷氨氮全局变量.vi" "状态告警区"() -> (w147:T4)
                  n86 = case shown="默认" w151 {
                    tunnel: [_ "总磷" ("table输入") "氨氮" ("table输入")] -> w149
                    frame Default {
                    }
                    frame 131 {
                    }
                    frame 92 {
                    }
                  }
                  n87 = Unbundle By Name(w147) -> ("F0"=w144:sgl, "F1"=w143:sgl, "F2"=w142:sgl, "F3"=w141:sgl, "id"=w140:u16, "flowid"=w139:u16, "量程"=w138:u16)
                  n88 = Format Into String(format string="F0=%04d,F1=%04d,F2=%0.4f,F3=%.04f,Flow=%d-%-d-%-d" ("格式字符串"), w144, w143, w142, w141, w140, w139, w138) -> (resulting string=w145:string)  [unwired: 2 in, 1 out]
                  n89 = Get Date/Time In Seconds() -> (seconds since 1Jan1904=w148:timestamp)
                  n90 = Bundle By Name(cluster=T10 {"时间标识"=timestamp(0 s since 1904-01-01), "设备"="", "日志信息"="", "流程参数"=""} ("data in"), "时间标识"=w148, "设备"=w149, "日志信息"=w132, "流程参数"=w145) -> (w150:T10)
                  n91 = call "总磷氨氮操作日志.vi"("data in"=w150) -> ()  [unwired: 11 in]
                }
              }
            }
            n92 = local write "数组"(w117) -> ()
          }
        }
      }
    }
    n93 = feedback #5() -> (w101:T9)  [unwired: 1 in]
    n94 = feedback-in #5(w85) -> ()
    n95 = Not Equal?(x=w85, y=w101) -> (x != y?=w102:cluster{"启动模式":bool, "启动参数":bool, "量程":bool})
    n96 = Cluster To Array(cluster=w102) -> (array=w103:bool[])
    n97 = Boolean Array To Number(Boolean array=w103) -> (number=w104:u32)
    n98 = Not Equal To 0?(x=w104) -> (x != 0?=w97:bool)
    n99 = First Call?() -> (First Call?: T/F=w98:bool)
    n100 = Or(x=w97, y=w98) -> (x .or. y?=w96:bool)
    n101 = while {
      tunnel: w96 -> [w242]
      tunnel: w85 -> [w241]
      shift-right: [w240] -> w100
      shift-left: _ -> [w236]
      shift-right: [w239] -> w99
      shift-left: _ -> [w237]
      stop <- TRUE stop-if-true
      n102 = case shown="真" w242 {
        tunnel: [w244 w251] -> w239
        tunnel: [w243 w250] -> w240
        tunnel: w241 -> [_ w245]
        tunnel: w237 -> [w244 _]
        tunnel: w236 -> [w243 _]
        frame False {
        }
        frame True {
          n103 = call "斯坦道XML解析.vi"("参数簇"=w245) -> ("步骤时间"=w246:string[], "步骤名"=w248:string[])  [unwired: 9 in]
          n104 = for {
            tunnel: w248 -> [_] mode=indexing
            tunnel: [w252] -> w249 mode=indexing
            i -> [w252]
          }
          n105 = Build Array(w248, w246) -> (w247:string[][])
          n106 = Transpose 2D Array(2D array=w247) -> (transposed array=w250:string[][])
          n107 = Number To Decimal String(number=w249) -> (decimal integer string=w251:string[])  [unwired: 1 in]
        }
      }
    }
    n108 = global read "VAR总磷氨氮全局变量.vi" "状态告警区"() -> (w86:T4)
    "总磷总氮运行状态" <- w86
    n109 = Unbundle By Name(w86) -> ("日志代码"=w73:u16)
    n110 = feedback-in #6(w73) -> ()
    n111 = feedback #6(w73) -> (w106:u16)
    n112 = Not Equal?(x=w73, y=w106) -> (x != y?=w105:bool)
    n113 = case shown="真" w105 {
      tunnel: w73 -> [_ w255]
      tunnel: w100 -> [_ w262]
      tunnel: w99 -> [_ w261]
      frame False {
      }
      frame True {
        n114 = Subtract(x=w255, y=1) -> (x-y=w253:i32)
        "多列列表框" <- w253
        n115 = Subtract(x=w253, y=5) -> (x-y=w257:i32)
        n116 = property on="多列列表框" class="MCListbox (严格)"("ItemNames"=w262, "RowHdrs[]"=w261) -> (error out=w263:errorcluster)  [unwired: 2 in, 1 out]
        n117 = Greater Or Equal To 0?(x=w257) -> (x >= 0?=w256:bool)
        n118 = property on="多列列表框" class="MCListbox (严格)"(error in=w263) -> (error out=w264:errorcluster, "TopLeft"=w265:T13)  [unwired: 1 in, 1 out]
        n119 = Select(t=w257, s=w256, f=0) -> (s? t:f=w258:i32)
        n120 = Bundle By Name(cluster=w265, "Row"=w258) -> (w266:T13)
        n121 = property on="多列列表框" class="MCListbox (严格)"(error in=w264, "TopLeft"=w266) -> ()  [unwired: 1 in, 2 out]
      }
    }
  }
  n122 = control-ref of="参数下拉列表"() -> (w13:refnum<vi>)
  n123 = control-ref of="量程下拉列表"() -> (w14:refnum<vi>)
  n124 = control-ref of="量程切换阈值"() -> (w10:refnum<vi>)
  n125 = node-c288() -> (w5:T14)  [unwired: 4 in]
  n126 = control-ref of="备用系数"() -> (w9:refnum<vi>)
  n127 = control-ref of="公式"() -> (w11:refnum<vi>)
  n128 = Obtain Queue(name (unnamed)="TP" ("名称（未命名）"), element data type=cluster{"命令":string, "data":variant} {"命令"="", "data"=variant}) -> (queue out=w34:refnum<queue>, error out=w35:errorcluster)  [unwired: 3 in, 1 out]
  n129 = property class="VI"(reference=w31) -> ("Name"=w30:string)  [unwired: 1 in, 2 out]
  n130 = timed-loop {
    timing: w5 -> [_]
    timing-out: [_] -> w4
    tunnel: w1 -> [w269]
    stop <- FALSE stop-if-true
    w270 = u16 3 items=["总磷"=1, "氨氮"=3] ("站号")
    # "定时更新"
    n131 = node-c288() -> ()  [unwired: 1 in, 1 out]
    n132 = call "总磷氨氮版本号读取.vi"() -> ("固件版本号"=→"固件版本号":string)  [unwired: 11 in]
    n133 = Bundle By Name(cluster=cluster{"命令":string, "data":variant} {"命令"="", "data"=variant} ("元素"), "命令"="读序列号", "data"=w270) -> (w268:cluster{"命令":string, "data":variant})
    n134 = Enqueue Element(queue=w269, element=w268) -> ()  [unwired: 2 in, 3 out]
    n135 = node-c288() -> ()  [unwired: 1 in, 1 out]
  }
  n136 = while {
    tunnel: w34 -> [w282]
    tunnel: w14 -> [w281]
    tunnel: w13 -> [w280]
    tunnel: w12 -> [w279]
    tunnel: w11 -> [w278]
    tunnel: w10 -> [w277]
    tunnel: w9 -> [w276]
    tunnel: w7 -> [_]
    stop <- FALSE stop-if-true
    n137 = event shown="[2] \"手动启动\": 值改变" {
      selector: _ -> [_ _ _ _ _ _ _ _ _ _ _ _ _ _ _ _]
      dyn-events: _ -> [_ _ _ _ _ _ _ _ _ _ _ _ _ _ _ _]
      timeout: _ -> [_ _ _ _ _ _ _ _ _ _ _ _ _ _ _ _]
      tunnel: w282 -> [_ _ w288 _ w299 w301 _ _ _ _ _ _ _ _ _ _]
      tunnel: w281 -> [_ _ _ _ _ _ _ _ _ _ w354 _ w374 w383 _ _]
      tunnel: w280 -> [_ _ _ _ _ _ _ _ _ _ w352 _ w372 w385 w393 w400]
      tunnel: w279 -> [_ _ _ _ _ _ _ _ _ _ w353 _ w373 w384 _ _]
      tunnel: w278 -> [_ _ _ _ _ _ _ _ _ _ w348 _ _ _ _ _]
      tunnel: w277 -> [_ _ _ _ _ _ _ _ _ _ _ _ w368 _ _ _]
      tunnel: w276 -> [_ _ _ _ _ _ _ _ _ _ _ _ _ _ w391 _]
      event Timeout {
        n138 = event-data() -> ()  [unwired: 1 in, 3 out]
      }
      event "同步时间": Value Change {
        n139 = event-data() -> ()  [unwired: 1 in, 6 out]
        n140 = call "总磷氨氮控制命令.vi"("参数"="参数") -> ("error out"=→"error out":errorcluster)  [unwired: 10 in]
      }
      event "手动启动": Value Change {
        n141 = event-data() -> ()  [unwired: 1 in, 6 out]
        n142 = call "总磷氨氮启动参数对话框.vi"() -> ("确认"=w286:bool, "元素"=w287:cluster{"命令":string, "data":variant})  [unwired: 10 in]
        n143 = case shown="真" w286 {
          tunnel: w288 -> [_ w290]
          tunnel: w287 -> [_ w289]
          frame False {
          }
          frame True {
            n144 = Enqueue Element(queue=w290, element=w289) -> ()  [unwired: 2 in, 3 out]
          }
        }
      }
      event "定时启动": Mouse Down {
        n145 = event-data() -> ()  [unwired: 1 in, 6 out]
        n146 = call "定时启动对话框.vi"() -> ("设置值"=→"设置值":dbl, "确定输出"=→"定时启动":bool)  [unwired: 10 in]
      }
      event "单步测试": Value Change {
        w294 = u16 1 items=["总磷"=1, "氨氮"=3] ("站号")
        n147 = event-data() -> ()  [unwired: 1 in, 6 out]
        n148 = Bundle("站号"=w294, "总磷氨氮调试"="总磷氨氮调试") -> (w293:cluster{"站号":u16, "总磷氨氮调试":u16[]})  [unwired: 1 in]
        n149 = Bundle By Name(cluster=cluster{"命令":string, "data":variant} {"命令"="", "data"=variant} ("元素"), "命令"="debug", "data"=w293) -> (w296:cluster{"命令":string, "data":variant})
        n150 = Enqueue Element(queue=w299, element=w296) -> ()  [unwired: 2 in, 3 out]
      }
      event "停止": Value Change {
        n151 = event-data() -> ()  [unwired: 1 in, 6 out]
        n152 = Enqueue Element(queue=w301, element=cluster{"命令":string, "data":variant} {"命令"="启动", "data"=variant(cluster{"站号":u16, "控制命令输出":u16[]} {"站号"=1, "控制命令输出"=[2816]})} ("元素")) -> ()  [unwired: 2 in, 3 out]
      }
      event "设置": Value Change {
        n153 = event-data() -> ()  [unwired: 1 in, 6 out]
        n154 = property on="窗格" class="Pane"("Origin"=T6 {"Horizontal"=0, "Vertical"=528} ("原点")) -> ()  [unwired: 2 in, 2 out]
      }
      event "返回": Value Change {
        n155 = event-data() -> ()  [unwired: 1 in, 6 out]
        n156 = property on="窗格" class="Pane"("Origin"=T6 {"Horizontal"=0, "Vertical"=0} ("原点")) -> ()  [unwired: 2 in, 2 out]
      }
      event "标液浓度1", "测量吸光度1", "测量吸光度2", "标液浓度2", "测量吸光度3", "标液浓度3", "测量吸光度4", "标液浓度4", "测量吸光度5", "标液浓度5", "样品1启用", "样品3启用", "样品4启用", "样品5启用", "样品2启用", "模型", "method", "样品1 F0", "样品1 F1", "样品2 F1", "样品2 F0", "样品3 F1", "样品4 F0", "样品4 F1", "样品5 F1", "样品5 F0", "精度": Value Change {
        n157 = event-data() -> ()  [unwired: 1 in, 6 out]
        n158 = formula code="E=log(F0/F1);"("F0"="样品1 F0", "F1"="样品1 F1") -> ("E"=w325:dbl)
        "测量吸光度1" <- w325
        n159 = formula code="E=log(F0/F1);"("F0"="样品2 F0", "F1"="样品2 F1") -> ("E"=w322:dbl)
        "测量吸光度2" <- w322
        n160 = formula code="E=log(F0/F1);"("F0"="样品3 F0", "F1"="样品3 F1") -> ("E"=w319:dbl)
        "测量吸光度3" <- w319
        n161 = formula code="E=log(F0/F1);"("F0"="样品4 F0", "F1"="样品4 F1") -> ("E"=w316:dbl)
        "测量吸光度4" <- w316
        n162 = formula code="E=log(F0/F1);"("F0"="样品5 F0", "F1"="样品5 F1") -> ("E"=w313:dbl)
        "测量吸光度5" <- w313
        n163 = Replace Array Subset(array=dbl[] [0.0, 0.0, 0.0, 0.0, 0.0] ("数组"), new element #1="标液浓度1", new element #2="标液浓度2", new element #3="标液浓度3", new element #4="标液浓度4", new element #5="标液浓度5") -> (w310:dbl[])  [unwired: 5 in]
        n164 = Replace Array Subset(array=dbl[] [0.0, 0.0, 0.0, 0.0, 0.0] ("数组"), new element #1=w325, new element #2=w322, new element #3=w319, new element #4=w316, new element #5=w313) -> (w309:dbl[])  [unwired: 5 in]
        n165 = Replace Array Subset(array=bool[] [FALSE, FALSE, FALSE, FALSE, FALSE] ("数组"), new element #1="样品1启用", new element #2="样品2启用", new element #3="样品3启用", new element #4="样品4启用", new element #5="样品5启用") -> (w308:bool[])  [unwired: 5 in]
        n166 = call "线性公式.vi"("精度"="精度", "模型"="模型", "method"="method", "启用"=w308, "监测浓度"=w309, "标液浓度"=w310) -> ("XY图"=→"XY图":cluster{"X Values":dbl[], "Y Values":dbl[]}[], "r^2"=→"r^2":dbl, "拟合方程"=→"拟合公式":string)  [unwired: 3 in]
      }
      event "标液浓度1", "标液浓度2", "标液浓度3", "标液浓度4", "标液浓度5", "样品1 F0", "样品1 F1", "样品2 F1", "样品2 F0", "样品3 F1", "样品3 F0", "样品4 F0", "样品4 F1", "样品5 F0", "样品5 F1", "精度", "公式.X^2", "公式.X", "公式.b", "量程切换阈值.阈值", "量程切换阈值.标液浓度", "备用系数.量程上限", "备用系数.量程下限", "备用系数.检出限", "备用系数.精度": Mouse Down {
        n167 = event-data() -> ("CtlRef"=w344:refnum<vi>)  [unwired: 1 in, 5 out]
        n168 = property class="DigNum (严格)"(reference=w344) -> (reference out=w342:refnum<vi>, "Value"=w343:dbl)  [unwired: 1 in, 1 out]
        n169 = call "数字键盘.vi"("OldNumber"=w343) -> ("NewNumber"=w341:sgl)
        n170 = property class="DigNum (严格)"(reference=w342, "Val(Sgnl)"=w341) -> ()  [unwired: 1 in, 2 out]
      }
      event "读公式": Value Change {
        n171 = event-data() -> ()  [unwired: 1 in, 6 out]
        n172 = property class="Enum (严格)"(reference=w352) -> ("Value"=w351:enum16{"氨氮"})  [unwired: 1 in, 2 out]
        n173 = property class="Enum (严格)"(reference=w353) -> ("Value"=w350:enum16{"水样测量", "空白核查", "标样核查", "盲样测试", "加标回收"})  [unwired: 1 in, 2 out]
        n174 = property class="Enum (严格)"(reference=w354) -> ("Value"=w349:enum16{"低量程", "高量程"})  [unwired: 1 in, 2 out]
        n175 = call "总磷氨氮公式读取.vi"("量程"=w349, "测量模式"=w350, "测量参数"=w351) -> ("error out"=w346:errorcluster, "公式"=w347:cluster{"X^2":dbl, "X":dbl, "b":dbl})  [unwired: 7 in]
        n176 = property class="Clust (严格)"(reference=w348, "Value"=w347) -> ()  [unwired: 1 in, 2 out]
        n177 = case shown="错误" w346 {
          tunnel: ["读取成功" ("消息") "读取失败" ("消息")] -> w345
          frame No Error {
          }
          frame Error {
          }
        }
        n178 = One Button Dialog(message=w345) -> ()  [unwired: 1 in, 1 out]
      }
      event "写公式": Value Change {
        n179 = event-data() -> ()  [unwired: 1 in, 6 out]
        n180 = call "总磷氨氮公式写入.vi"("公式"="公式", "量程"="量程下拉列表", "测量模式"="测量模式下拉列表", "测量参数"="参数下拉列表") -> ("error out"=w357:errorcluster)  [unwired: 7 in]
        n181 = case shown="无错误" w357 {
          tunnel: ["写入成功" ("消息") "写入失败" ("消息")] -> w358
          frame No Error {
          }
          frame Error {
          }
        }
        n182 = One Button Dialog(message=w358) -> ()  [unwired: 1 in, 1 out]
      }
      event "量程切换阈值读取": Value Change {
        n183 = event-data() -> ()  [unwired: 1 in, 6 out]
        n184 = property class="Enum (严格)"(reference=w372) -> ("Value"=w371:enum16{"氨氮"})  [unwired: 1 in, 2 out]
        n185 = property class="Enum (严格)"(reference=w373) -> ("Value"=w370:enum16{"水样测量", "空白核查", "标样核查", "盲样测试", "加标回收"})  [unwired: 1 in, 2 out]
        n186 = property class="Enum (严格)"(reference=w374) -> ("Value"=w369:enum16{"低量程", "高量程"})  [unwired: 1 in, 2 out]
        n187 = call "总磷氨氮量程读取.vi"("量程"=w369, "测量模式"=w370, "测量参数"=w371) -> ("error out"=w365:errorcluster, "量程切换阈值"=w367:cluster{"阈值":dbl, "标液浓度":dbl})  [unwired: 7 in]
        n188 = property class="Clust (严格)"(reference=w368, "Value"=w367) -> ()  [unwired: 1 in, 2 out]
        n189 = case shown="错误" w365 {
          tunnel: ["读取成功" ("消息") "读取失败" ("消息")] -> w366
          frame No Error {
          }
          frame Error {
          }
        }
        n190 = One Button Dialog(message=w366) -> ()  [unwired: 1 in, 1 out]
      }
      event "量程切换阈值写入": Value Change {
        n191 = event-data() -> ()  [unwired: 1 in, 6 out]
        n192 = property class="Enum (严格)"(reference=w385) -> ("Value"=w382:enum16{"氨氮"})  [unwired: 1 in, 2 out]
        n193 = property class="Enum (严格)"(reference=w384) -> ("Value"=w381:enum16{"水样测量", "空白核查", "标样核查", "盲样测试", "加标回收"})  [unwired: 1 in, 2 out]
        n194 = property class="Enum (严格)"(reference=w383) -> ("Value"=w380:enum16{"低量程", "高量程"})  [unwired: 1 in, 2 out]
        n195 = call "总磷氨氮量程写入.vi"("量程切换阈值"="量程切换阈值", "量程"=w380, "测量模式"=w381, "测量参数"=w382) -> ("error out"=w377:errorcluster)  [unwired: 7 in]
        n196 = case shown="无错误" w377 {
          tunnel: ["写入成功" ("消息") "写入失败" ("消息")] -> w378
          frame No Error {
          }
          frame Error {
          }
        }
        n197 = One Button Dialog(message=w378) -> ()  [unwired: 1 in, 1 out]
      }
      event "备用系数读取": Value Change {
        n198 = event-data() -> ()  [unwired: 1 in, 6 out]
        n199 = property class="Enum (严格)"(reference=w393) -> ("Value"=w392:enum16{"氨氮"})  [unwired: 1 in, 2 out]
        n200 = call "总磷氨氮备用系数读取.vi"("测量参数"=w392) -> ("error out"=w388:errorcluster, "备用系数"=w390:T2)  [unwired: 9 in]
        n201 = property class="Clust (严格)"(reference=w391, "Value"=w390) -> ()  [unwired: 1 in, 2 out]
        n202 = case shown="错误" w388 {
          tunnel: ["读取成功" ("消息") "读取失败" ("消息")] -> w389
          frame No Error {
          }
          frame Error {
          }
        }
        n203 = One Button Dialog(message=w389) -> ()  [unwired: 1 in, 1 out]
      }
      event "备用系数写入": Value Change {
        n204 = event-data() -> ()  [unwired: 1 in, 6 out]
        n205 = property class="Enum (严格)"(reference=w400) -> ("Value"=w399:enum16{"氨氮"})  [unwired: 1 in, 2 out]
        n206 = call "总磷氨氮备用系数写入.vi"("备用系数"="备用系数", "测量参数"=w399) -> ("error out"=w396:errorcluster)  [unwired: 9 in]
        n207 = case shown="无错误" w396 {
          tunnel: ["写入成功" ("消息") "写入失败" ("消息")] -> w397
          frame No Error {
          }
          frame Error {
          }
        }
        n208 = One Button Dialog(message=w397) -> ()  [unwired: 1 in, 1 out]
      }
    }
  }
  n209 = property class="VI"(reference=w23) -> ("Name"=w16:string)  [unwired: 1 in, 2 out]
  n210 = while {
    tunnel: w34 -> [w405]
    shift-right: [w406] -> _
    shift-left: T5."待机" -> [w407]
    shift-right: [w403] -> _
    shift-left: u32 0 ("等待时间（毫秒）") -> [w404]
    stop <- FALSE stop-if-true
    n211 = Wait (ms)(milliseconds to wait=u32 1000 ("等待时间（毫秒）")) -> ()  [unwired: 1 out]
    n212 = local read "定时启动"() -> (w408:bool)
    n213 = case shown="真" w408 {
      tunnel: w407 -> [_ w416]
      tunnel: [T5."待机" w415] -> w406
      tunnel: w405 -> [_ w414]
      tunnel: w404 -> [_ w413]
      tunnel: [_ w412] -> w403
      frame False {
      }
      frame True {
        n214 = case shown="\"待机\", 默认" w416 {
          tunnel: [w417 w429 w436 w447 w455 w467] -> w415
          tunnel: w414 -> [_ w434 _ w453 _ _]
          tunnel: w413 -> [_ _ _ _ _ w470]
          tunnel: [_ _ _ _ _ w466] -> w412
          frame "待机", Default {
            n215 = global read "VAR总磷氨氮全局变量.vi" "状态告警区"() -> (w420:T4)
            n216 = Unbundle By Name(w420) -> ("工作状态"=w418:T8, "id"=w419:u16)
            n217 = case shown="默认" w418 {
              tunnel: w419 -> [_ w423]
              tunnel: [T5."启动氨氮" w422] -> w417
              frame "空闲" {
              }
              frame Default {
                n218 = case shown="131, 默认" w423 {
                  tunnel: [T5."启动氨氮" T5."启动总磷"] -> w422
                  frame 92 {
                  }
                  frame 131, Default {
                  }
                }
              }
            }
          }
          frame "启动氨氮" {
            n219 = call "总磷氨氮启动命令.vi"("参数"=T17 {"站号"=3, "量程切换"=enum."AUTO", "控制命令"=enum."启动测量", "模式设置"=enum."待机", "测量间隔"=0}) -> ("启动命令"=w427:cluster{"命令":string, "data":variant})  [unwired: 10 in]
            n220 = Enqueue Element(queue=w434, element=w427) -> ()  [unwired: 2 in, 3 out]
            n221 = global read "VAR总磷氨氮全局变量.vi" "状态告警区"() -> (w433:T4)
            n222 = Unbundle By Name(w433) -> ("工作状态"=w432:T8)
            n223 = Not Equal To 0?(x=w432) -> (x != 0?=w431:bool)
            n224 = Select(t=T5."氨氮测量中", s=w431, f=T5."启动氨氮") -> (s? t:f=w429:T5)
          }
          frame "氨氮测量中" {
            n225 = flat-sequence {
              tunnel: [w440] -> w435
              tunnel: [w444] -> w436
              tunnel: w435 -> [w444]
              frame #0 {
                n226 = global read "VAR总磷氨氮全局变量.vi" "状态告警区"() -> (w441:T4)
                n227 = Unbundle By Name(w441) -> ("工作状态"=w442:T8)
                n228 = Equal To 0?(x=w442) -> (x = 0?=w438:bool)
                n229 = Select(t=T5."延时", s=w438, f=T5."氨氮测量中") -> (s? t:f=w440:T5)
              }
              frame #1 {
                n230 = Wait (ms)(milliseconds to wait=u32 5000 ("等待时间（毫秒）")) -> ()  [unwired: 1 out]
              }
            }
          }
          frame "启动总磷" {
            n231 = call "总磷氨氮启动命令.vi"("参数"=T17 {"站号"=1, "量程切换"=enum."AUTO", "控制命令"=enum."启动测量", "模式设置"=enum."待机", "测量间隔"=0}) -> ("启动命令"=w446:cluster{"命令":string, "data":variant})  [unwired: 10 in]
            n232 = Enqueue Element(queue=w453, element=w446) -> ()  [unwired: 2 in, 3 out]
            n233 = global read "VAR总磷氨氮全局变量.vi" "状态告警区"() -> (w448:T4)
            n234 = Unbundle By Name(w448) -> ("工作状态"=w449:T8)
            n235 = Not Equal To 0?(x=w449) -> (x != 0?=w450:bool)
            n236 = Select(t=T5."总磷测量中", s=w450, f=T5."启动总磷") -> (s? t:f=w447:T5)
          }
          frame "总磷测量中" {
            n237 = flat-sequence {
              tunnel: [w457] -> w454
              tunnel: [w463] -> w455
              tunnel: w454 -> [w463]
              frame #0 {
                n238 = global read "VAR总磷氨氮全局变量.vi" "状态告警区"() -> (w460:T4)
                n239 = Unbundle By Name(w460) -> ("工作状态"=w461:T8)
                n240 = Equal To 0?(x=w461) -> (x = 0?=w456:bool)
                n241 = Select(t=T5."延时", s=w456, f=T5."总磷测量中") -> (s? t:f=w457:T5)
              }
              frame #1 {
                n242 = Wait (ms)(milliseconds to wait=u32 5000 ("等待时间（毫秒）")) -> ()  [unwired: 1 out]
              }
            }
          }
          frame "延时" {
            n243 = local read "设置值"() -> (w469:dbl)
            n244 = Increment(x=w470) -> (x+1=w466:u32)
            n245 = Greater Or Equal?(x=w466, y=w469) -> (x >= y?=w468:bool)
            n246 = Select(t=T5."待机", s=w468, f=T5."延时") -> (s? t:f=w467:T5)
          }
        }
      }
    }
  }
  n247 = while {
    tunnel: w34 -> [w479]
    tunnel: w35 -> [_]
    shift-right: [w471] -> _
    shift-left: enum16{"氨氮", "总磷"}."氨氮" ("枚举") -> [w473]
    stop <- FALSE stop-if-true
    # "试剂填充 172 \n管路清洗108\n氨氮92\n总磷131\n总磷海水147\n总氮76\n总氮海水92"
    n248 = case shown="\"氨氮\", 默认" w473 {
      selector: w473 -> [w485 w487]
      tunnel: [w486 w488] -> w474
      tunnel: [w485 w487] -> w472
      frame "氨氮", Default {
        w486 = u16 3 items=["总磷"=1, "氨氮"=3] ("站号")
      }
      frame "总磷" {
        w488 = u16 1 items=["总磷"=1, "氨氮"=3] ("站号")
      }
    }
    n249 = Wait (ms)(milliseconds to wait=u32 1000 ("等待时间（毫秒）")) -> ()  [unwired: 1 out]
    n250 = Bundle By Name(cluster=cluster{"命令":string, "data":variant} {"命令"="", "data"=variant} ("元素"), "命令"="读状态告警区", "data"=w474) -> (w481:cluster{"命令":string, "data":variant})
    n251 = Enqueue Element(queue=w479, element=w481) -> (queue out=w475:refnum<queue>)  [unwired: 2 in, 2 out]
    n252 = Increment(x=w472) -> (x+1=w471:enum16{"氨氮", "总磷"})
    n253 = Bundle By Name(cluster=cluster{"命令":string, "data":variant} {"命令"="", "data"=variant} ("元素"), "命令"="读测量数据区", "data"=w474) -> (w477:cluster{"命令":string, "data":variant})
    n254 = Enqueue Element(queue=w475, element=w477) -> ()  [unwired: 2 in, 3 out]
  }
  n255 = Open VI Reference(type specifier VI Refnum (for type only)=refnum<vi> refnum, vi path=w30, options=128 ("选项")) -> (vi reference=w28:refnum<vi>, error out=w26:errorcluster)  [unwired: 3 in]
  n256 = call-by-ref "?"(reference=w28, error in=w26) -> (reference out=w24:refnum<vi>, error out=w25:errorcluster)  [unwired: 12 in]
  n257 = Open VI Reference(type specifier VI Refnum (for type only)=refnum<vi> refnum, vi path=w16, options=128 ("选项")) -> (vi reference=w18:refnum<vi>, error out=w20:errorcluster)  [unwired: 3 in]
  n258 = call-by-ref "?"(reference=w18, error in=w20) -> (reference out=w22:refnum<vi>, error out=w21:errorcluster)  [unwired: 12 in]
  n259 = Close Reference(reference=w24, error in (no error)=w25) -> ()  [unwired: 1 out]
  n260 = Close Reference(reference=w22, error in (no error)=w21) -> ()  [unwired: 1 out]
  n261 = node-c288(w4) -> ()  [unwired: 1 out]
